vi "bit_address.vi"(8 "Min time SCL Low":u32 caption="Count(uSec)", 9 "Min time SCL High":u32 caption="Count(uSec)", 10 "Read /write":bool, 11 "Address":u32) -> ()   [LabVIEW 2019]
uses:
  <vilib>/rvi/eio/common/nirviEmuTemplateMethod_errors.vi
  <vilib>/eio/EIONode/EIONode.xnode
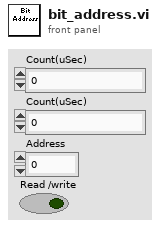
[diagram p1: front panel]
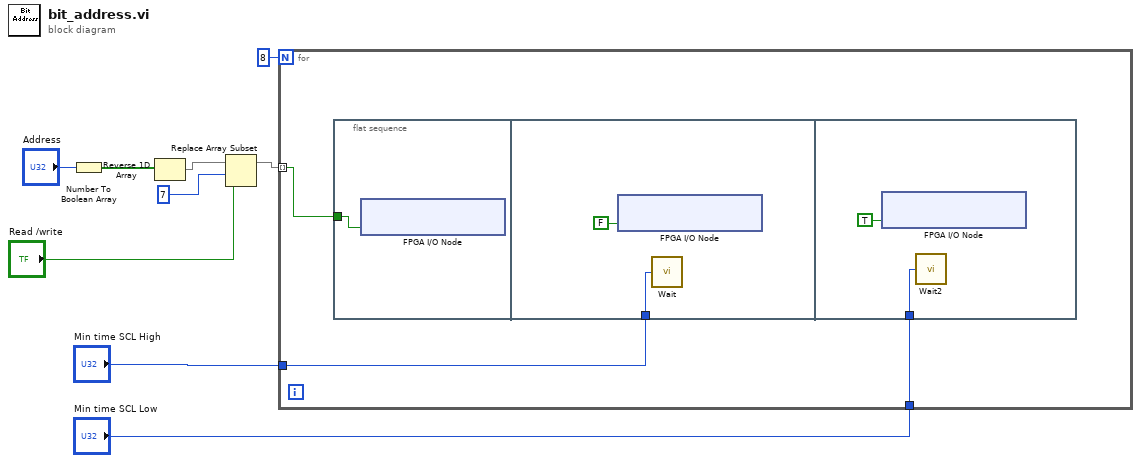
[diagram p0: block diagram]
diagram:
  n1 = Number To Boolean Array(number="Address") -> (Boolean array=w9:bool[])
  n2 = Reverse 1D Array(array=w9) -> (reversed array=w8:bool[])
  n3 = Replace Array Subset(array=w8, new element="Read /write", index=7) -> (w7:bool[])
  n4 = for {
    N: 8 -> [_]
    tunnel: w7 -> [w12] mode=indexing
    tunnel: "Min time SCL High" -> [w11]
    tunnel: "Min time SCL Low" -> [w10]
    n5 = flat-sequence {
      tunnel: w12 -> [w13]
      tunnel: w11 -> [w14]
      tunnel: w10 -> [w16]
      frame #0 {
        n6 = xnode "FPGA I/O Node"("ConnectorA/DIO15"=w13) -> ()  [unwired: 1 in, 1 out]
      }
      frame #1 {
        n7 = xnode "FPGA I/O Node"("ConnectorA/DIO14"=FALSE) -> ()  [unwired: 1 in, 1 out]
        n8 = call "Wait"("Count(uSec)"=w14) -> ()  [unwired: 1 out]
      }
      frame #2 {
        n9 = xnode "FPGA I/O Node"("ConnectorA/DIO14"=TRUE) -> ()  [unwired: 1 in, 1 out]
        n10 = call "Wait2"("Count(uSec)"=w16) -> ()  [unwired: 1 out]
      }
    }
  }
